vi "Main page.vi"() -> ()   [LabVIEW 2020]
uses:
  Port details.ctl
  SM Cases.ctl
  Control Pages.ctl
  Data Acquisition.ctl
  Array of Port Config.ctl
  Global Data Cluster.ctl
panel:
  out "Proc loop time":dbl
  out "Status":string
  in  "left arrow":bool
  in  "right arrow":bool
  in  "Refresh":bool
  in  "Logout":bool
  out "error out":errorcluster
  in  "Error In":errorcluster
  in  "Instructions":bool
  out "Tab Control":T1(tab)
  out "Success":string
  in  "Confirm":bool
  in  "New Password":string
  in  "Current Password":string
  out "login text":string
  in  "Change password":bool
  in  "Delete User":bool
  in  "View users":bool
  in  "Add user":bool
  in  "Logout user":bool
  in  "Password":string
  in  "Signin":bool
  in  "User Name":string
  in  "Channel2":T2={"Port No."="", "Checkbox"=FALSE, "Parity"=0, "Stop Bit"=0, "Baud Rate"=9600, "Data Bits"=8} {"Stop Bit" items=["1.0", "1.5", "2.0"]; "Parity" items=["None", "Odd", "Even", "Mark", "Space"]}
  in  "Channel1":T3={"Port No."="", "Checkbox"=FALSE, "Parity"=0, "Stop Bit"=0, "Baud Rate"=9600, "Data Bits"=8} {"Stop Bit" items=["1.0", "1.5", "2.0"]; "Parity" items=["None", "Odd", "Even", "Mark", "Space"]}
  in  "Channel8":T2={"Port No."="", "Checkbox"=FALSE, "Parity"=0, "Stop Bit"=0, "Baud Rate"=9600, "Data Bits"=8} {"Stop Bit" items=["1.0", "1.5", "2.0"]; "Parity" items=["None", "Odd", "Even", "Mark", "Space"]}
  in  "Channel7":T2={"Port No."="", "Checkbox"=FALSE, "Parity"=0, "Stop Bit"=0, "Baud Rate"=9600, "Data Bits"=8} {"Stop Bit" items=["1.0", "1.5", "2.0"]; "Parity" items=["None", "Odd", "Even", "Mark", "Space"]}
  in  "Channel6":T2={"Port No."="", "Checkbox"=FALSE, "Parity"=0, "Stop Bit"=0, "Baud Rate"=9600, "Data Bits"=8} {"Stop Bit" items=["1.0", "1.5", "2.0"]; "Parity" items=["None", "Odd", "Even", "Mark", "Space"]}
  in  "Channel5":T2={"Port No."="", "Checkbox"=FALSE, "Parity"=0, "Stop Bit"=0, "Baud Rate"=9600, "Data Bits"=8} {"Stop Bit" items=["1.0", "1.5", "2.0"]; "Parity" items=["None", "Odd", "Even", "Mark", "Space"]}
  in  "Channel4":T2={"Port No."="", "Checkbox"=FALSE, "Parity"=0, "Stop Bit"=0, "Baud Rate"=9600, "Data Bits"=8} {"Stop Bit" items=["1.0", "1.5", "2.0"]; "Parity" items=["None", "Odd", "Even", "Mark", "Space"]}
  in  "Channel3":T2={"Port No."="", "Checkbox"=FALSE, "Parity"=0, "Stop Bit"=0, "Baud Rate"=9600, "Data Bits"=8} {"Stop Bit" items=["1.0", "1.5", "2.0"]; "Parity" items=["None", "Odd", "Even", "Mark", "Space"]}
  in  "Cancel Config":bool
  in  "Save":bool
  in  "Config file view":bool
  out "File Name":string
  in  "Multicolumn Listbox":i32[](listbox)
  in  "Cancel Frame Config":bool
  in  "Save file":bool
  in  "New File":bool
  in  "View data":bool
  in  "Edit structure":bool
  in  "Remove structure":bool
  in  "Add structure":bool
  out "Version":string
  in  "EOH":u8 format="%x"
  in  "No. of bytes":u16 format="%x"
  in  "Message ID":u8 format="%x"
  in  "SOH":u8 format="%x"
  in  "Channel name":u16(ring) items=["Channel1", "Channel2", "Channel3", "Channel4", "Channel5", "Channel6", "Channel7", "Channel8"]
  in  "Cancel Acq":bool
  in  "Stop Acquisition":bool
  in  "Start Acquisition":bool
  in  "FCS Configuration":u16(ring) items=["6012", "7210", "Data_Structure ", "Sim_Struct ", "Sim_Struct_1Port ", "Sim_Struct_3Ports ", "Struct_Channel3 ", "V7352"]
  in  "Port Configuration":u16(ring) items=["LRU_1Port ", "LRU_ch1&2 ", "LRU_ch3&4 ", "LRU_Channel3 ", "LRU_Channel_Config ", "LRU_Config_3Ports ", "LRU_Port_Config "]
  out "% Failure 3":dbl
  out "CRC Failure 3":u32
  out "Frames Read 3":u32
  out "Channel 3":u8(slide) scale=0.0..100.0
  out "% Failure 8":dbl
  out "CRC Failure 8":u32
  out "Frames Read 8":u32
  out "Channel 8":u8(slide) scale=0.0..100.0
  out "% Failure 7":dbl
  out "CRC Failure 7":u32
  out "Frames Read 7":u32
  out "Channel 7":u8(slide) scale=0.0..100.0
  out "% Failure 6":dbl
  out "CRC Failure 6":u32
  out "Frames Read 6":u32
  out "Channel 6":u8(slide) scale=0.0..100.0
  out "% Failure 5":dbl
  out "CRC Failure 5":u32
  out "Frames Read 5":u32
  out "Channel 5":u8(slide) scale=0.0..100.0
  out "% Failure 4":dbl
  out "CRC Failure 4":u32
  out "Frames Read 4":u32
  out "Channel 4":u8(slide) scale=0.0..100.0
  out "% Failure 2":dbl
  out "CRC Failure 2":u32
  out "Frames Read 2":u32
  out "Channel 2":u8(slide) max=150 scale=0.0..100.0
  out "% Failure":dbl
  out "CRC Failure":u32
  out "Frames Read":u32
  out "Channel 1":u8(slide) max=150 scale=0.0..100.0
  in  "Log CRC Failure":enum32{"Log File Yes", "Log File No"}(radio)=enum."Log File No"
  in  "Done":bool
  in  "Refresh":bool
  in  "Update":bool
  in  "Data File Type":enum32{"bin type", "txt type"}(radio)=enum."txt type"
  in  "Data Folder Path":path=path "C:/Users/BEL/Desktop/FCS Rx Data"
  in  "Data Structure Folder Path":path=path "D:/BEL_FCS_Project/FCTS_JIG_LV/Configuration Files/Data Structure"
  in  "Configuration Folder Path":path=path "D:/BEL_FCS_Project/FCTS_JIG_LV/Configuration Files/Port Configuration"
  in  "Help":bool
  in  "Information":bool
  in  "Configuration":bool
  in  "Frame Info":bool
  in  "Frame Format":bool
  in  "Port Configuration":bool
  in  "Authentication":bool
  # "FLIGHT CONTROL SYSTEM\nTEST JIG"
  # "Change Password"
  # "Delete User"
  # "Logout"
  # "Add User"
  # "View Users"
  # "BHARAT ELECTRONICS"
  # "FLIGHT CONTROL SYSTEM (FCS) \nTEST JIG"
  # "COMAVIA SYSTEMS TECHNOLOGIES PRIVATE LIMITED"
  # "VERSION NO."
  # "1.0.0"
  # "RELEASED DATE:"
  # "30/06/2020"
  # "DEVELOPED BY:"
  # "Serial Configuration"
  # "Frame Format"
  # "EOH"
  # "Message ID"
  # "No. of Bytes"
  # "Channel"
  # "SOH"
  # "Frame Info"
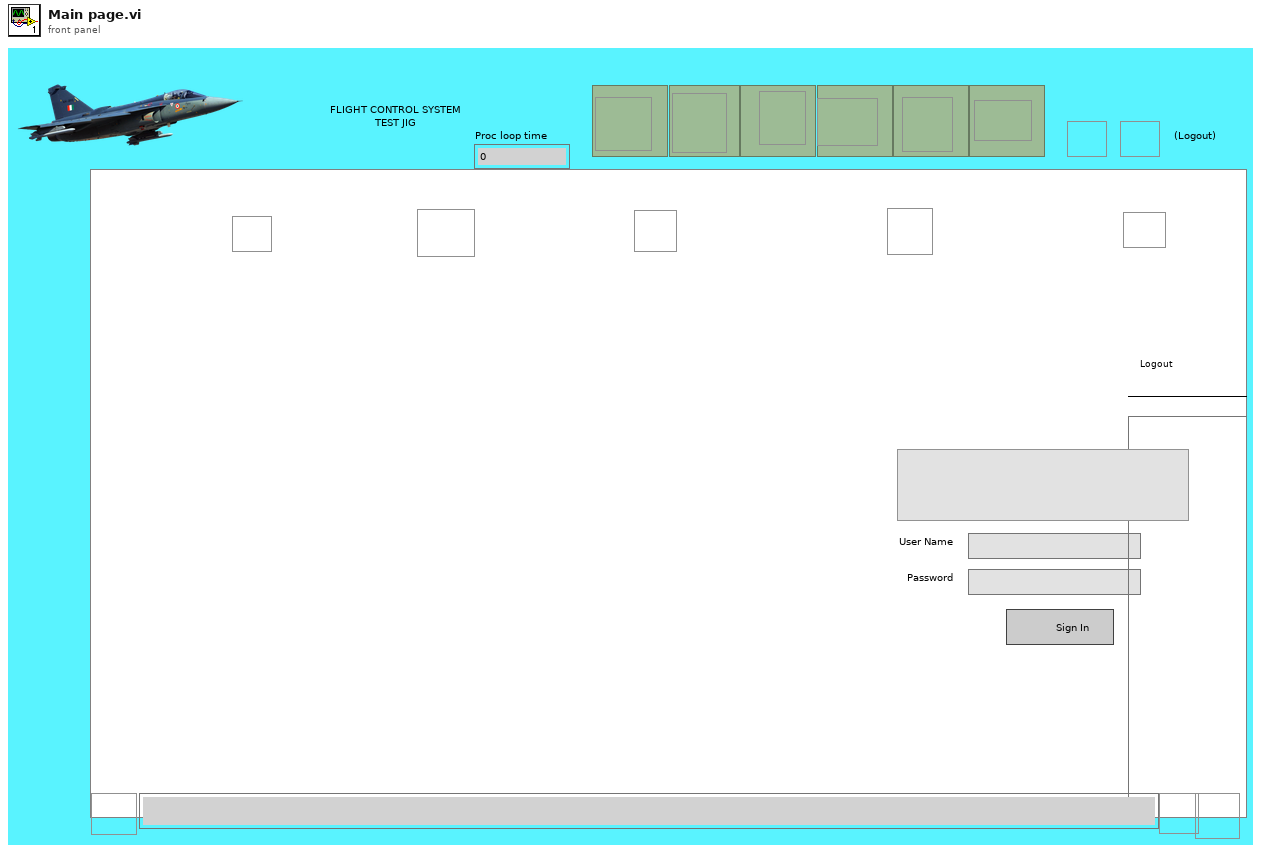
[diagram p1: front panel]
types:
  T1 = enum32{"Authentication", "Home", "Port Config", "Frame Format", "Frame Info", "Configuration", "Page 6", "Page 7"}
  T2 = typedef "Port details.ctl" = cluster{"Port No.":refnum<visa-resource-name>, "Checkbox":bool, "Parity":u16, "Stop Bit":u16, "Baud Rate":u32, "Data Bits":u8}
  T3 = cluster{"Port No.":refnum<visa-resource-name>, "Checkbox":bool, "Parity":u16, "Stop Bit":u16, "Baud Rate":u32, "Data Bits":u8}
  T4 = typedef "SM Cases.ctl" = enum32{"Self-Test", "Initialize", "Poll", "Authentication", "Port Config", "Frame Format", "Frame Info", "Configuration", "User Info", "Logout", "Exit"}
  T5 = typedef "Control Pages.ctl" = enum32{"Authentication", "Home", "Port Config", "Frame Format", "Frame Info", "Configuration", "Page 6", "Page 7"}
  T6 = enum8{"Enabled", "Disabled", "Disabled and Grayed Out"}
  T7 = typedef "Global Data Cluster.ctl" = cluster{"log paths":path[], "CRC paths":path[], "log refnum":refnum<file>[], "CRC refnum":refnum<file>[], "unfiltered array":string[], "Port config":cluster{"data":cluster{"Port No.":refnum<visa-resource-name>, "Checkbox":bool, "Parity":u16, "Stop Bit":u16, "Baud Rate":u32, "Data Bits":u8}[]}, "Filtered array":string[], "Data Structure":string[][]}
  T8 = typedef "Array of Port Config.ctl" = cluster{"Port No.":refnum<visa-resource-name>, "Checkbox":bool, "Parity":u16, "Stop Bit":u16, "Baud Rate":u32, "Data Bits":u8}[]
  T9 = typedef "Data Acquisition.ctl" = enum16{"Port Config", "File Open", "Process Data", "Data Logging", "File Close", "Exit"}
  T10 = enum16{"big-endian, network order", "native, host order", "little-endian"}
  T11 = enum16{"open", "replace", "create", "open or create", "replace or create", "replace or create with confirmation"}
  T12 = cluster{"Port No.":refnum<visa-resource-name>, "Checkbox":bool, "Parity":u16, "Stop Bit":u16, "Baud Rate":u32, "Data Bits":u8}[]
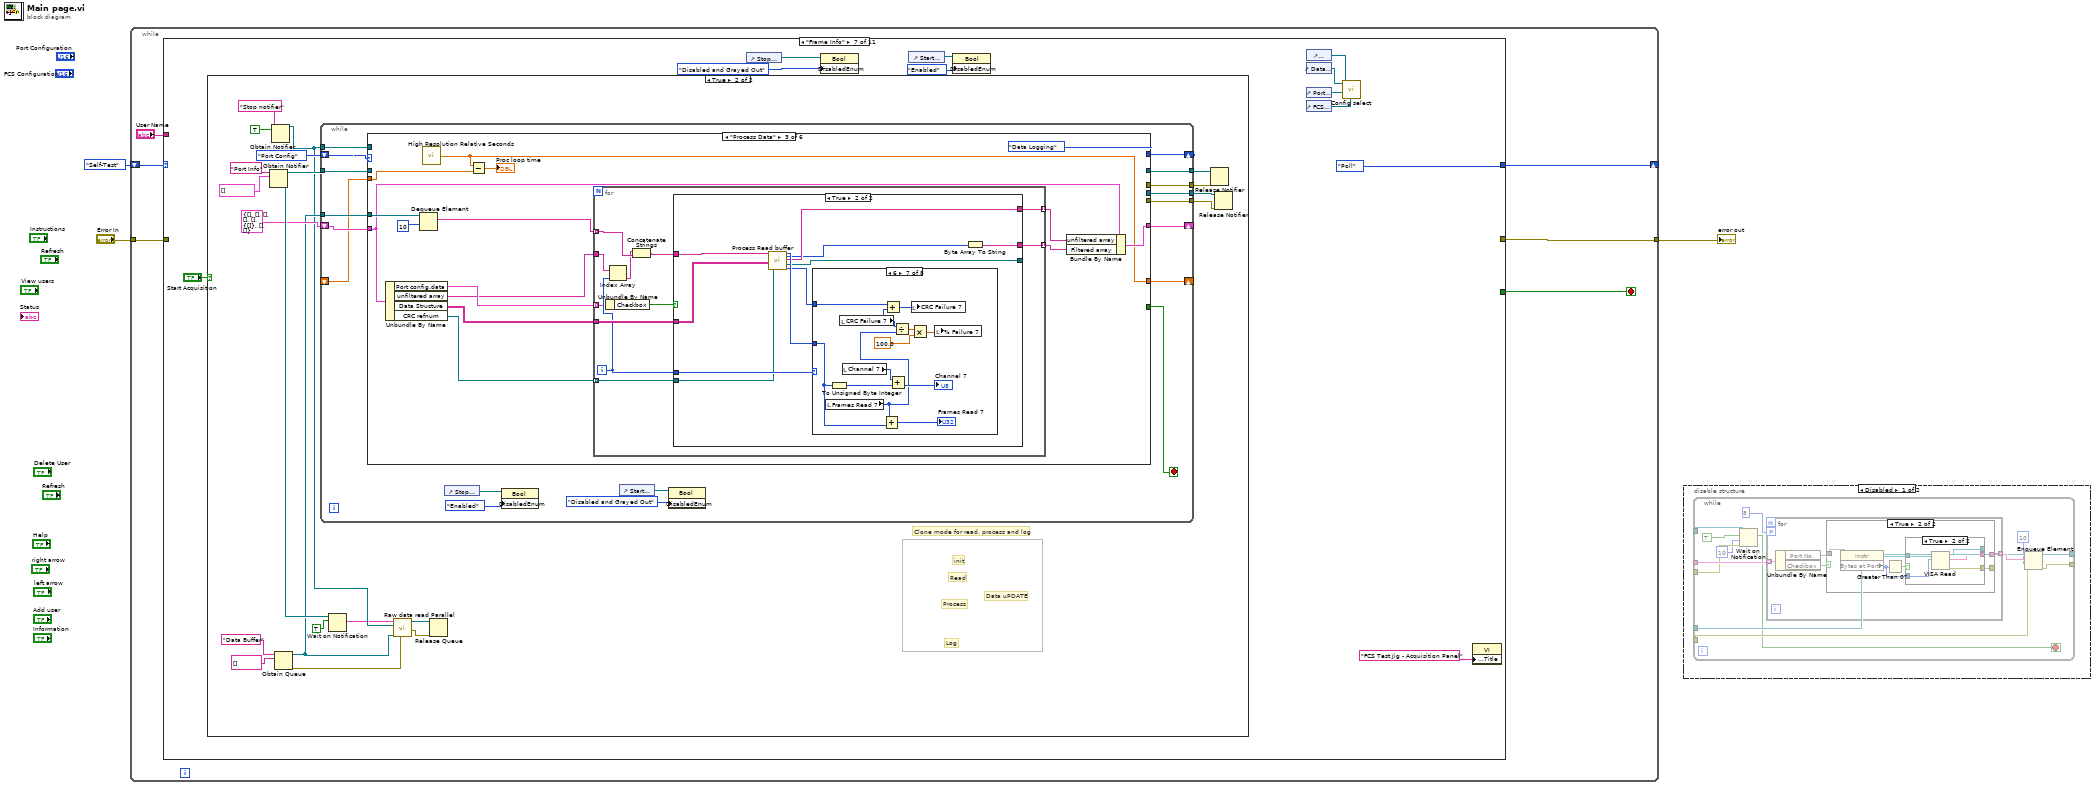
[diagram p0: block diagram]
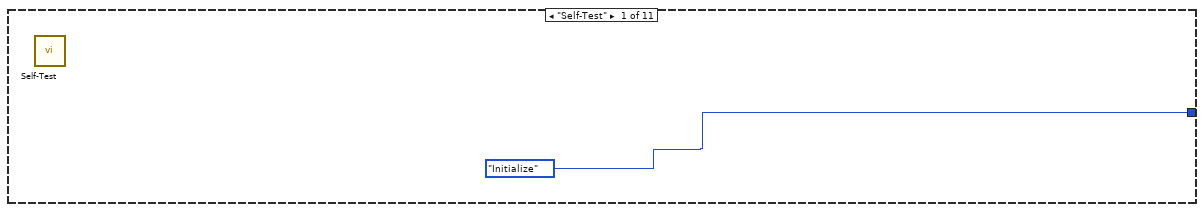
[diagram p5: hidden frame]
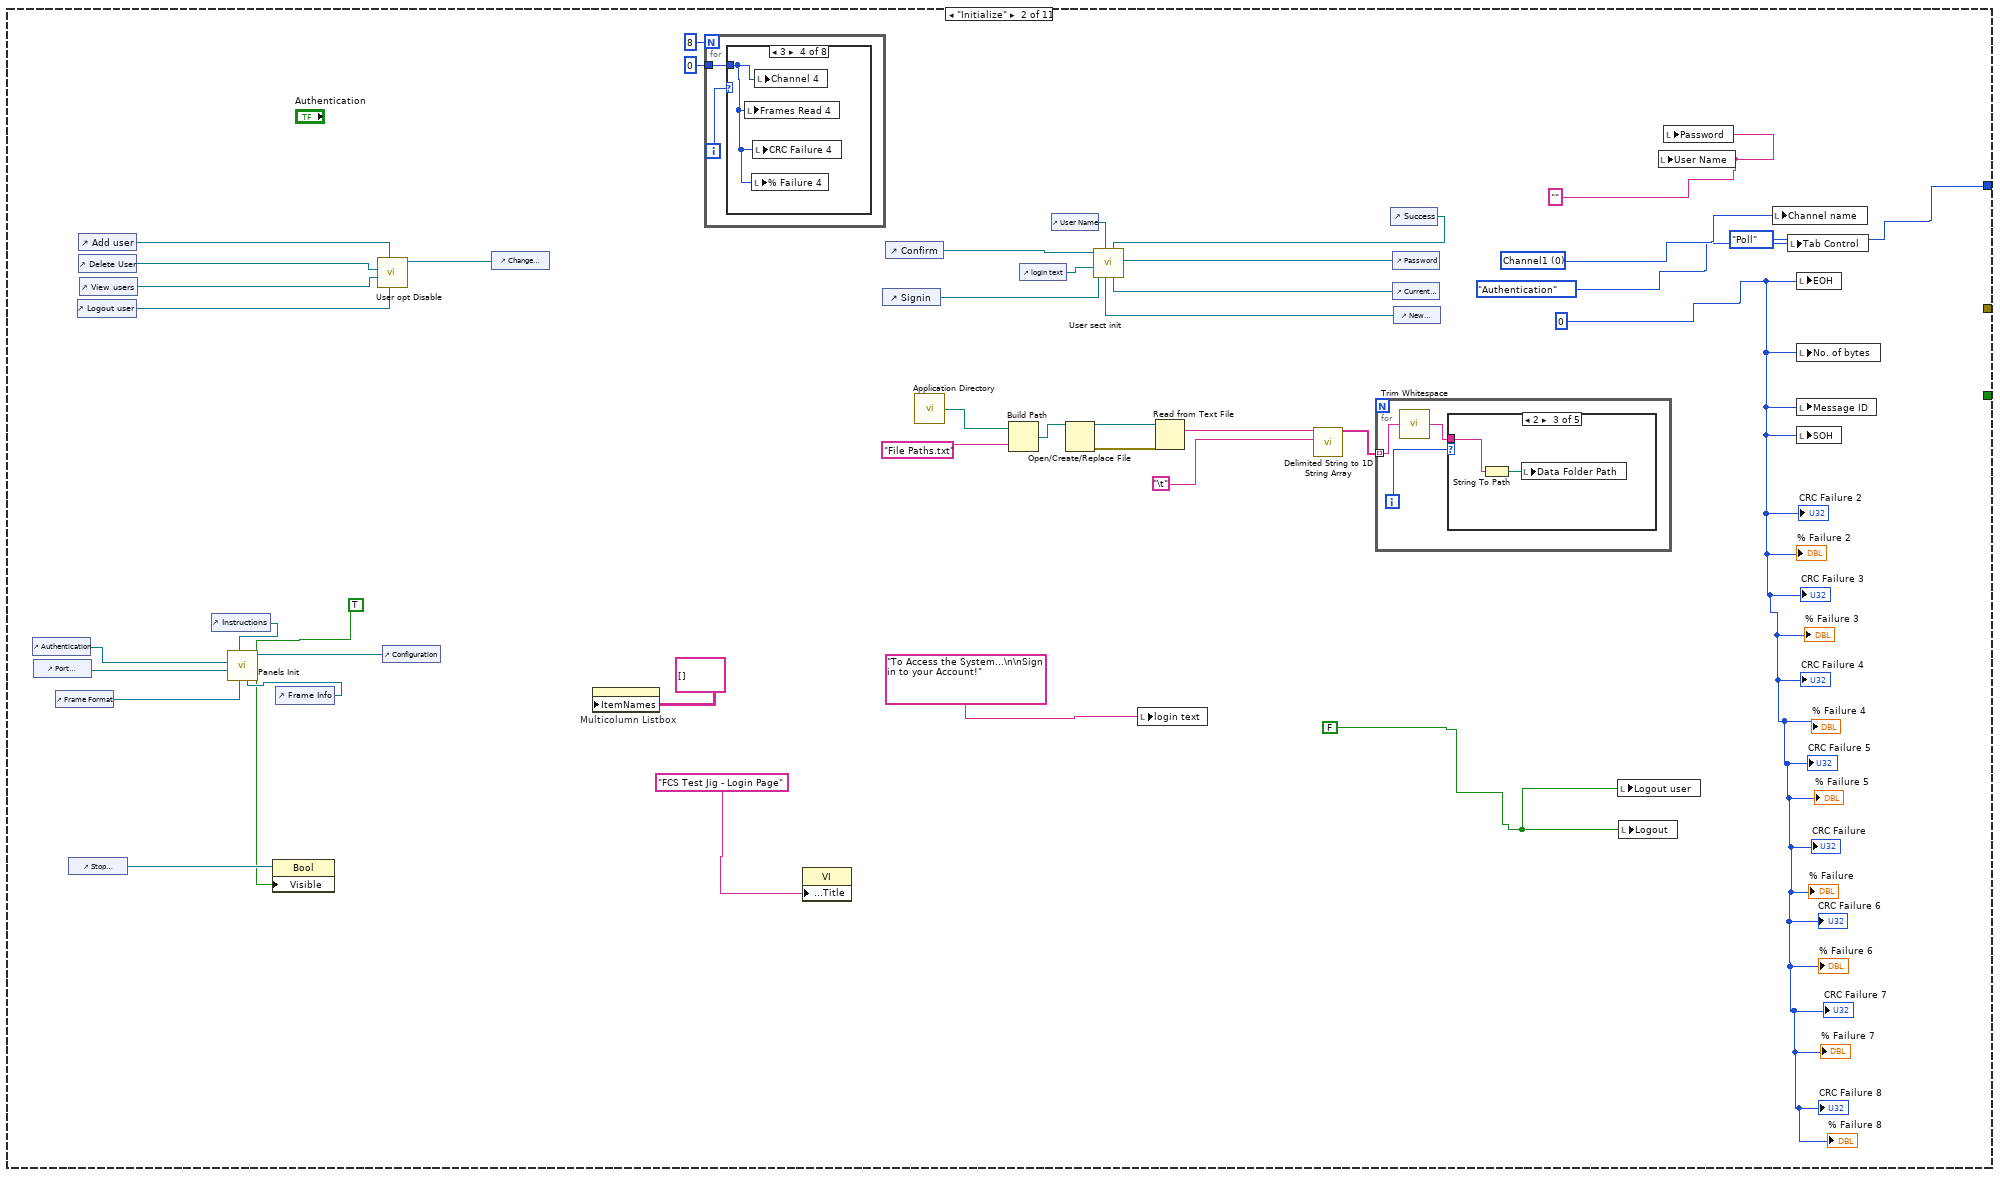
[diagram p6: hidden frame]
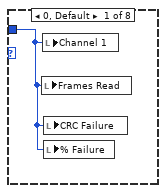
[diagram p7: hidden frame]
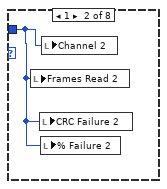
[diagram p8: hidden frame]
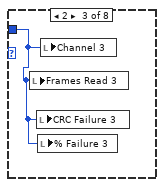
[diagram p9: hidden frame]
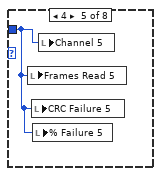
[diagram p10: hidden frame]
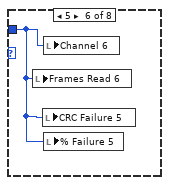
[diagram p11: hidden frame]
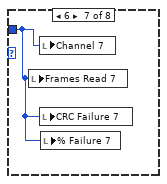
[diagram p12: hidden frame]
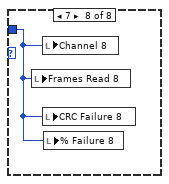
[diagram p13: hidden frame]
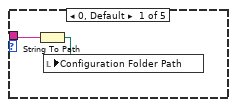
[diagram p14: hidden frame]
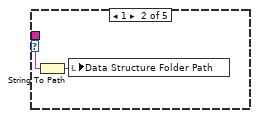
[diagram p15: hidden frame]
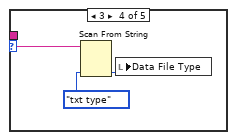
[diagram p16: hidden frame]
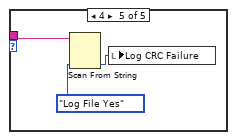
[diagram p17: hidden frame]
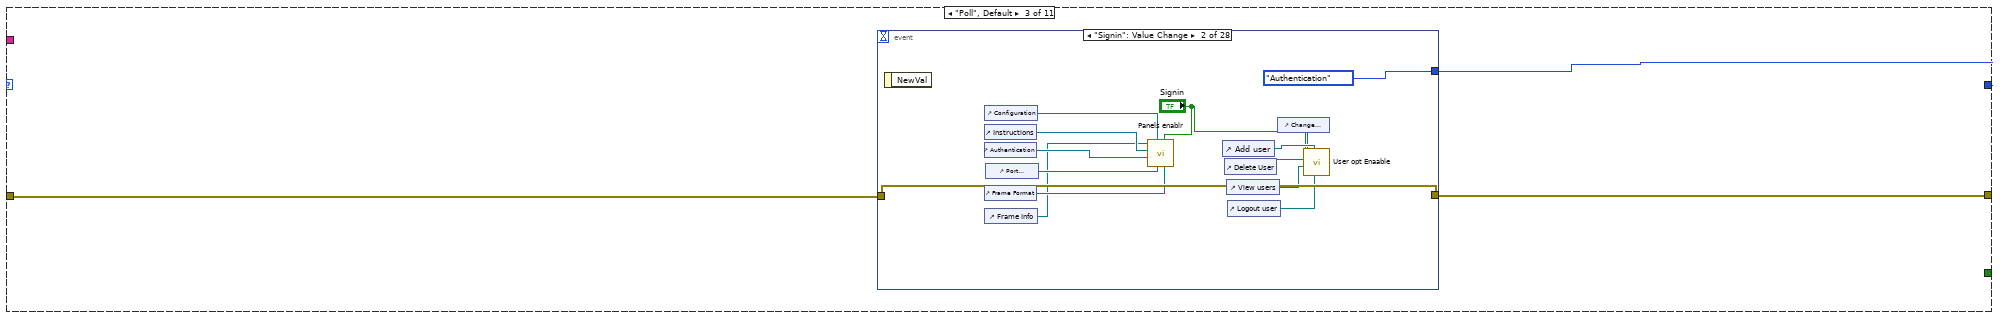
[diagram p18: hidden frame]
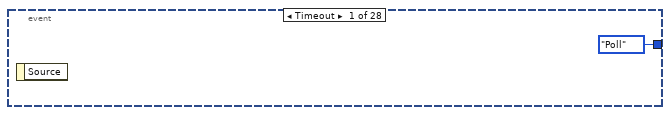
[diagram p19: hidden frame]
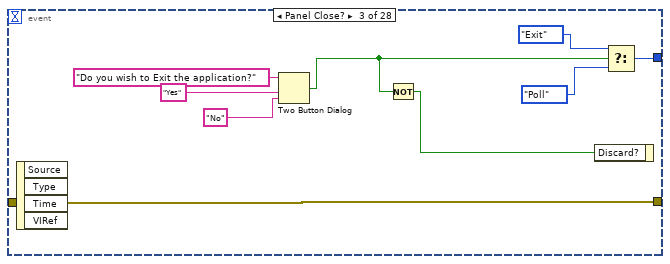
[diagram p20: hidden frame]
diagram:
  n1 = while {
    tunnel: "Error In" -> [w8]
    tunnel: [w7] -> w2
    shift-right: [w6] -> _
    shift-left: SM_Cases."Self-Test" ("Tab Control") -> [w9]
    stop <- w5 stop-if-true
    n2 = case shown="\"Frame Info\"" w9 {
      tunnel: [_ _ w78 w152 _ _ _ _ _ _ _] -> w7
      tunnel: w8 -> [_ _ w77 w153 _ _ _ w567 _ _ _]
      tunnel: [SM_Cases."Initialize" ("Tab Control") SM_Cases."Poll" ("Tab Control") w76 SM_Cases."Poll" ("Tab Control") SM_Cases."Poll" ("Tab Control") SM_Cases."Poll" ("Tab Control") SM_Cases."Poll" ("Tab Control") SM_Cases."Poll" ("Tab Control") SM_Cases."Poll" ("Tab Control") SM_Cases."Initialize" ("Tab Control") SM_Cases."Poll" ("Tab Control")] -> w6
      tunnel: [_ _ _ _ _ _ _ _ _ _ TRUE] -> w5
      tunnel: "User Name" -> [_ _ _ w148 _ _ _ _ _ w629 _]
      frame "Self-Test" {
        n3 = call "Self-Test.vi"() -> ()  [unwired: 12 in]
      }
      frame "Initialize" {
        w11 = FALSE ("Logout")
        w14 = u32 0 ("EOH")
        w49 = u16 0 items=["Channel1", "Channel2", "Channel3", "Channel4", "Channel5", "Channel6", "Channel7", "Channel8"] ("Ring")
        w29 = "" ("Password")
        n4 = control-ref of="Authentication"() -> (w41:refnum<vi>)
        n5 = control-ref of="Port Configuration"() -> (w40:refnum<vi>)
        n6 = control-ref of="Frame Format"() -> (w39:refnum<vi>)
        n7 = control-ref of="Stop Acquisition"() -> (w24:refnum<vi>)
        n8 = control-ref of="Logout user"() -> (w32:refnum<vi>)
        n9 = control-ref of="Add user"() -> (w33:refnum<vi>)
        n10 = control-ref of="Delete User"() -> (w34:refnum<vi>)
        n11 = control-ref of="View users"() -> (w35:refnum<vi>)
        n12 = control-ref of="Instructions"() -> (w36:refnum<vi>)
        n13 = property class="Bool"(reference=w24, "Visible"=TRUE) -> ()  [unwired: 1 in, 2 out]
        n14 = control-ref of="Frame Info"() -> (w38:refnum<vi>)
        n15 = control-ref of="Configuration"() -> (w37:refnum<vi>)
        n16 = call "Panels Init.vi"("Frame Info"=w38, "Frame Format"=w39, "Instructions"=w36, "Port Configuration"=w40, "Authentication"=w41, "Boolean in"=w37) -> ()  [unwired: 6 in]
        n17 = control-ref of="Change password"() -> (w31:refnum<vi>)
        n18 = call "User opt Disable.vi"("Logout user"=w32, "Add user"=w33, "View users"=w35, "Delete User"=w34, "Boolean in"=w31) -> ()  [unwired: 7 in]
        n19 = property on="Multicolumn Listbox" class="MCListbox (strict)"("ItemNames"=string[][] [] ("Item Names")) -> ()  [unwired: 2 in, 2 out]
        n20 = for {
          N: 8 -> [_]
          tunnel: u32 0 -> [w52]
          i -> [w51]
          n21 = case shown="3" w51 {
            tunnel: w52 -> [w53 w54 w55 w56 w57 w58 w59 w60]
            frame 0, Default {
              n22 = local write "Frames Read"(w53) -> ()
              n23 = local write "Channel 1"(w53) -> ()
              n24 = local write "CRC Failure"(w53) -> ()
              n25 = local write "% Failure"(w53) -> ()
            }
            frame 1 {
              n26 = local write "Frames Read 2"(w54) -> ()
              n27 = local write "CRC Failure 2"(w54) -> ()
              n28 = local write "% Failure 2"(w54) -> ()
              n29 = local write "Channel 2"(w54) -> ()
            }
            frame 2 {
              n30 = local write "Frames Read 3"(w55) -> ()
              n31 = local write "CRC Failure 3"(w55) -> ()
              n32 = local write "% Failure 3"(w55) -> ()
              n33 = local write "Channel 3"(w55) -> ()
            }
            frame 3 {
              n34 = local write "Frames Read 4"(w56) -> ()
              n35 = local write "% Failure 4"(w56) -> ()
              n36 = local write "CRC Failure 4"(w56) -> ()
              n37 = local write "Channel 4"(w56) -> ()
            }
            frame 4 {
              n38 = local write "Frames Read 5"(w57) -> ()
              n39 = local write "CRC Failure 5"(w57) -> ()
              n40 = local write "% Failure 5"(w57) -> ()
              n41 = local write "Channel 5"(w57) -> ()
            }
            frame 5 {
              n42 = local write "Frames Read 6"(w58) -> ()
              n43 = local write "CRC Failure 5"(w58) -> ()
              n44 = local write "Channel 6"(w58) -> ()
              n45 = local write "% Failure 5"(w58) -> ()
            }
            frame 6 {
              n46 = local write "Frames Read 7"(w59) -> ()
              n47 = local write "Channel 7"(w59) -> ()
              n48 = local write "CRC Failure 7"(w59) -> ()
              n49 = local write "% Failure 7"(w59) -> ()
            }
            frame 7 {
              n50 = local write "Frames Read 8"(w60) -> ()
              n51 = local write "Channel 8"(w60) -> ()
              n52 = local write "CRC Failure 8"(w60) -> ()
              n53 = local write "% Failure 8"(w60) -> ()
            }
          }
        }
        n54 = property class="VI"("Front Panel.Title"="FCS Test Jig - Login Page" ("VI Name")) -> ()  [unwired: 2 in, 2 out]
        n55 = control-ref of="Signin"() -> (w46:refnum<vi>)
        n56 = control-ref of="Confirm"() -> (w44:refnum<vi>)
        n57 = call <vilib>:"Application Directory.vi"() -> ("Application Directory"=w22:path)
        n58 = Build Path(base path=w22, name or relative path="File Paths.txt") -> (appended path=w20:path)
        n59 = control-ref of="login text"() -> (w47:refnum<vi>)
        n60 = control-ref of="User Name"() -> (w28:refnum<vi>)
        n61 = Open/Create/Replace File(file path (use dialog)=w20) -> (refnum out=w18:refnum<file>, error out=w19:errorcluster)  [unwired: 5 in, 1 out]
        n62 = local write "login text"("To Access the System...\n\nSign in to your Account!" ("login text")) -> ()
        n63 = Read from Text File(file (use dialog)=w18, error in=w19) -> (text=w17:string)  [unwired: 2 in, 3 out]
        n64 = call <vilib>:"Delimited String to 1D String Array.vi"("delimiter"="\t", "delimited string"=w17) -> ("string array"=w15:string[])  [unwired: 9 in]
        n65 = for {
          tunnel: w15 -> [w62] mode=indexing
          i -> [w63]
          n66 = call <vilib>:"Trim Whitespace.vi"("string"=w62) -> ("trimmed string"=w61:string)  [unwired: 1 in]
          n67 = case shown="2" w63 {
            tunnel: w61 -> [w65 w67 w69 w72 w75]
            frame 0, Default {
              n68 = String To Path(string=w65) -> (path=w64:path)
              n69 = local write "Configuration Folder Path"(w64) -> ()
            }
            frame 1 {
              n70 = String To Path(string=w67) -> (path=w66:path)
              n71 = local write "Data Structure Folder Path"(w66) -> ()
            }
            frame 2 {
              n72 = String To Path(string=w69) -> (path=w68:path)
              n73 = local write "Data Folder Path"(w68) -> ()
            }
            frame 3 {
              n74 = Scan From String(input string=w72, default 1=enum32{"bin type", "txt type"}."txt type" ("Data File Type")) -> (output 1=w70:enum32{"bin type", "txt type"})  [unwired: 3 in, 3 out]
              n75 = local write "Data File Type"(w70) -> ()
            }
            frame 4 {
              n76 = Scan From String(input string=w75, default 1=enum32{"Log File Yes", "Log File No"}."Log File Yes" ("Log CRC Failure")) -> (output 1=w73:enum32{"Log File Yes", "Log File No"})  [unwired: 3 in, 3 out]
              n77 = local write "Log CRC Failure"(w73) -> ()
            }
          }
        }
        n78 = control-ref of="Success"() -> (w42:refnum<vi>)
        n79 = control-ref of="Password"() -> (w48:refnum<vi>)
        n80 = control-ref of="Current Password"() -> (w45:refnum<vi>)
        n81 = control-ref of="New Password"() -> (w43:refnum<vi>)
        n82 = call "User sect init.vi"("Current Password"=w45, "Success"=w42, "New Password"=w43, "User Name"=w28, "Signin"=w46, "login text"=w47, "Password"=w48, "Boolean in"=w44) -> ()  [unwired: 4 in]
        n83 = local write "Logout user"(w11) -> ()
        n84 = local write "Logout"(w11) -> ()
        n85 = local write "User Name"(w29) -> ()
        n86 = local write "Password"(w29) -> ()
        n87 = local write "Channel name"(w49) -> ()
        n88 = local write "Tab Control"(Control_Pages."Authentication" ("Tab Control")) -> ()
        n89 = local write "EOH"(w14) -> ()
        n90 = local write "No. of bytes"(w14) -> ()
        n91 = local write "Message ID"(w14) -> ()
        n92 = local write "SOH"(w14) -> ()
        "CRC Failure 2" <- w14
        "% Failure 2" <- w14
        "CRC Failure 3" <- w14
        "% Failure 3" <- w14
        "CRC Failure 4" <- w14
        "% Failure 4" <- w14
        "CRC Failure 5" <- w14
        "% Failure 5" <- w14
        "CRC Failure 6" <- w14
        "% Failure 6" <- w14
        "CRC Failure 7" <- w14
        "% Failure 7" <- w14
        "CRC Failure 8" <- w14
        "% Failure 8" <- w14
        "CRC Failure" <- w14
        "% Failure" <- w14
      }
      frame "Poll", Default {
        n93 = event shown="[1] \"Signin\": Value Change" {
          selector: _ -> [_ _ _ _ _ _ _ _ _ _ _ _ _ _ _ _ _ _ _ _ _ _ _ _ _ _ _ _]
          dyn-events: _ -> [_ _ _ _ _ _ _ _ _ _ _ _ _ _ _ _ _ _ _ _ _ _ _ _ _ _ _ _]
          timeout: _ -> [_ _ _ _ _ _ _ _ _ _ _ _ _ _ _ _ _ _ _ _ _ _ _ _ _ _ _ _]
          tunnel: [_ w93 w102 _ _ _ _ _ _ _ _ _ _ _ _ _ _ _ _ _ _ _ _ _ _ _ _ _] -> w78
          tunnel: w77 -> [_ w93 w102 _ _ _ _ _ _ _ _ _ _ _ _ _ _ _ _ _ _ _ _ _ _ _ _ _]
          tunnel: [SM_Cases."Poll" ("Tab Control") SM_Cases."Authentication" ("Tab Control") w97 SM_Cases."Frame Format" ("Tab Control") SM_Cases."Port Config" ("Tab Control") SM_Cases."Frame Info" ("Tab Control") SM_Cases."User Info" ("Tab Control") SM_Cases."Logout" ("Tab Control") SM_Cases."User Info" ("Tab Control") SM_Cases."User Info" ("Tab Control") SM_Cases."Logout" ("Tab Control") SM_Cases."Port Config" ("Tab Control") SM_Cases."Configuration" ("Tab Control") SM_Cases."Configuration" ("Tab Control") SM_Cases."Frame Format" ("Tab Control") SM_Cases."Frame Format" ("Tab Control") SM_Cases."Frame Format" ("Tab Control") SM_Cases."Frame Format" ("Tab Control") SM_Cases."Poll" ("Tab Control") SM_Cases."Port Config" ("Tab Control") SM_Cases."Frame Format" ("Tab Control") SM_Cases."Frame Format" ("Tab Control") SM_Cases."Poll" ("Tab Control") SM_Cases."Port Config" ("Tab Control") SM_Cases."Frame Format" ("Tab Control") SM_Cases."Frame Info" ("Tab Control") SM_Cases."Frame Info" ("Tab Control") SM_Cases."Configuration" ("Tab Control")] -> w76
          event Timeout {
            n94 = event-data() -> ()  [unwired: 1 in, 1 out]
          }
          event "Signin": Value Change {
            n95 = event-data() -> ()  [unwired: 1 in, 1 out]
            n96 = control-ref of="Instructions"() -> (w90:refnum<vi>)
            n97 = control-ref of="Authentication"() -> (w89:refnum<vi>)
            n98 = control-ref of="Frame Format"() -> (w87:refnum<vi>)
            n99 = control-ref of="Configuration"() -> (w91:refnum<vi>)
            n100 = control-ref of="Frame Info"() -> (w86:refnum<vi>)
            n101 = control-ref of="Port Configuration"() -> (w88:refnum<vi>)
            n102 = call "Panels enablr.vi"("Frame Format"=w87, "Signin"="Signin", "Port Configuration"=w88, "Configuration"=w91, "Authentication"=w89, "Instructions"=w90, "Boolean in"=w86) -> ()  [unwired: 5 in]
            n103 = control-ref of="Add user"() -> (w85:refnum<vi>)
            n104 = control-ref of="Delete User"() -> (w84:refnum<vi>)
            n105 = control-ref of="View users"() -> (w83:refnum<vi>)
            n106 = control-ref of="Logout user"() -> (w82:refnum<vi>)
            n107 = control-ref of="Change password"() -> (w81:refnum<vi>)
            n108 = call "User opt Enaable.vi"("Logout user"=w82, "Add user"=w85, "Boolean"="Signin", "View users"=w83, "Delete User"=w84, "Boolean in"=w81) -> ()  [unwired: 6 in]
          }
          event Panel Close? {
            n109 = event-data() -> ()  [unwired: 1 in, 4 out]
            n110 = Two Button Dialog(message="Do you wish to Exit the application?", 1:"No" ("F button name (\"Cancel\")"), 2:"Yes" ("T button name (\"OK\")")) -> (T button?=w95:bool)
            n111 = Not(x=w95) -> (.not. x?=w94:bool)
            n112 = event-data("Discard?"=w94) -> ()  [unwired: 1 in, 1 out]
            n113 = Select(t=SM_Cases."Exit" ("Tab Control"), s=w95, f=SM_Cases."Poll" ("Tab Control")) -> (s? t:f=w97:T4)
          }
          event "Frame Format": Value Change {
            n114 = event-data() -> ()  [unwired: 1 in, 1 out]
            n115 = local write "Tab Control"(T1."Frame Format" ("Tab Control")) -> ()
            n116 = local write "No. of bytes"(u16 1 ("No. of bytes")) -> ()
            n117 = local write "Message ID"(u8 1 ("Message ID")) -> ()
            n118 = local write "SOH"(u8 1 ("SOH")) -> ()
            n119 = local write "EOH"(u8 1 ("EOH")) -> ()
          }
          event "Port Configuration": Value Change {
            n120 = event-data() -> ()  [unwired: 1 in, 1 out]
            n121 = local write "Tab Control"(T1."Port Config" ("Tab Control")) -> ()
          }
          event "Frame Info": Value Change {
            n122 = event-data() -> ()  [unwired: 1 in, 1 out]
            n123 = local write "Tab Control"(T1."Frame Info" ("Tab Control")) -> ()
          }
          event "Authentication": Value Change {
            n124 = event-data() -> ()  [unwired: 1 in, 1 out]
            n125 = property class="VI"("Front Panel.Title"="FCS Test Jig - Access Panel" ("VI Name")) -> ()  [unwired: 2 in, 2 out]
            "Tab Control" <- T1."Authentication" ("Tab Control")
          }
          event "Logout user": Value Change {
            n126 = event-data() -> ()  [unwired: 1 in, 6 out]
          }
          event "Change password": Value Change {
            n127 = event-data() -> ()  [unwired: 1 in, 1 out]
          }
          event "Confirm": Value Change {
            n128 = event-data() -> ()  [unwired: 1 in, 6 out]
          }
          event "Logout": Value Change {
            n129 = event-data() -> ()  [unwired: 1 in, 6 out]
          }
          event "Save": Value Change {
            n130 = event-data() -> ()  [unwired: 1 in, 6 out]
          }
          event "Configuration": Value Change {
            n131 = event-data() -> ()  [unwired: 1 in, 6 out]
            n132 = local write "Tab Control"(T1."Configuration" ("Tab Control")) -> ()
          }
          event "Done": Value Change {
            n133 = event-data() -> ()  [unwired: 1 in, 6 out]
          }
          event "Add structure": Value Change {
            n134 = event-data() -> ()  [unwired: 1 in, 6 out]
          }
          event "Remove structure": Value Change {
            n135 = event-data() -> ()  [unwired: 1 in, 1 out]
          }
          event "Edit structure": Value Change {
            n136 = event-data() -> ()  [unwired: 1 in, 6 out]
          }
          event "Save file": Value Change {
            n137 = event-data() -> ()  [unwired: 1 in, 6 out]
          }
          event "Multicolumn Listbox": Double Click {
            n138 = event-data() -> ("Row"=w128:i32)  [unwired: 1 in]
            n139 = control-ref of="Multicolumn Listbox"() -> (w129:refnum<vi>)
            n140 = control-ref of="SOH"() -> (w133:refnum<vi>)
            n141 = control-ref of="Message ID"() -> (w132:refnum<vi>)
            n142 = control-ref of="No. of bytes"() -> (w131:refnum<vi>)
            n143 = control-ref of="EOH"() -> (w130:refnum<vi>)
            n144 = control-ref of="Channel name"() -> (w134:refnum<vi>)
            n145 = call "Structure Data Change.vi"("reference 5"=w130, "Row"=w128, "reference 4"=w131, "reference"=w134, "reference 3"=w132, "reference 2"=w133, "MCListbox Refnum"=w129) -> ()  [unwired: 5 in]
          }
          event "Config file view": Value Change {
            n146 = event-data() -> ()  [unwired: 1 in, 6 out]
          }
          event "View data": Value Change {
            n147 = event-data() -> ()  [unwired: 1 in, 6 out]
          }
          event "New File": Value Change {
            n148 = event-data() -> ()  [unwired: 1 in, 6 out]
          }
          event "Cancel Acq": Value Change {
            n149 = event-data() -> ()  [unwired: 1 in, 6 out]
            n150 = case shown="True" "Cancel Acq" {
              frame False {
              }
              frame True {
                n151 = local write "Tab Control"(T1."Home" ("Tab Control")) -> ()
                n152 = property class="VI"("Front Panel.Title"="FCS Test Jig - Home Page" ("VI Name")) -> ()  [unwired: 2 in, 2 out]
              }
            }
          }
          event "Cancel Config": Value Change {
            n153 = event-data() -> ()  [unwired: 1 in, 6 out]
          }
          event "Cancel Frame Config": Value Change {
            n154 = event-data() -> ()  [unwired: 1 in, 6 out]
          }
          event "Start Acquisition": Value Change {
            n155 = event-data() -> ()  [unwired: 1 in, 6 out]
          }
          event "Stop Acquisition": Value Change {
            n156 = event-data() -> ()  [unwired: 1 in, 6 out]
          }
          event "Update": Value Change {
            n157 = event-data() -> ()  [unwired: 1 in, 6 out]
          }
        }
      }
      frame "Authentication" {
        n158 = control-ref of="Tab Control"() -> (w150:refnum<vi>)
        n159 = control-ref of="Status"() -> (w151:refnum<vi>)
        n160 = call "User Authentication.vi"("User Name"=w148, "error in (no error)"=w153, "Password"="Password", "Status"=w151, "TabControl in"=w150) -> ("error out"=w152:errorcluster, "login text"=→"login text":string)  [unwired: 5 in]
      }
      frame "Port Config" {
        n161 = control-ref of="Channel7"() -> (w160:refnum<vi>)
        n162 = control-ref of="Channel2"() -> (w163:refnum<vi>)
        n163 = control-ref of="Channel8"() -> (w161:refnum<vi>)
        n164 = control-ref of="Configuration Folder Path"() -> (w164:refnum<vi>)
        n165 = control-ref of="Channel3"() -> (w162:refnum<vi>)
        n166 = control-ref of="Channel4"() -> (w159:refnum<vi>)
        n167 = control-ref of="Status"() -> (w179:refnum<vi>)
        n168 = local read "Configuration Folder Path"() -> (w178:path)
        n169 = call "Config File Save.vi"("String in"=w179, "Channel 5"="Channel5", "Channel 6"="Channel6", "Channel 7"="Channel7", "Channel 8"="Channel8", "Channel 1"="Channel1", "Configuration Folder Path"=w178, "Channel 4"="Channel4", "Channel 2"="Channel2", "Channel 3"="Channel3", "Save"="Save") -> ("File Name"=w168:string)  [unwired: 4 in]
        n170 = local write "File Name"(w168) -> ()
        n171 = control-ref of="Channel1"() -> (w166:refnum<vi>)
        n172 = control-ref of="Channel5"() -> (w158:refnum<vi>)
        n173 = control-ref of="Channel6"() -> (w157:refnum<vi>)
        n174 = call "File View SubVI.vi"("Channel 8"=w161, "Channel 1"=w166, "Config Path"=w164, "Config file view"="Config file view", "Channel 7"=w160, "Channel 2"=w163, "Channel 3"=w162, "Channel 4"=w159, "Channel 5"=w158, "Channel 6"=w157) -> ("File Name"=→"File Name":string)  [unwired: 5 in]
        n175 = case shown="True" "Cancel Config" {
          frame False {
          }
          frame True {
            n176 = local write "Tab Control"(T1."Home" ("Tab Control")) -> ()
            n177 = property class="VI"("Front Panel.Title"="FCS Test Jig - Home Page" ("VI Name")) -> ()  [unwired: 2 in, 2 out]
          }
        }
        n178 = property class="VI"("Front Panel.Title"="FCS Test Jig - Configuration Panel" ("VI Name")) -> ()  [unwired: 2 in, 2 out]
      }
      frame "Frame Format" {
        n179 = control-ref of="Multicolumn Listbox"() -> (w201:refnum<vi>)
        n180 = local read "Message ID"() -> (w198:u8)
        n181 = case shown="True" "New File" {
          frame False {
          }
          frame True {
            n182 = Initialize Array("") -> (w214:string[][])  [unwired: 2 in]
            n183 = property on="Multicolumn Listbox" class="MCListbox (strict)"("ItemNames"=w214) -> ()  [unwired: 2 in, 2 out]
          }
        }
        n184 = call "Add Structure.vi"("EOH"="EOH", "No. of bytes"="No. of bytes", 7:"Channel name", "MCListbox Refnum"=w201, "Message ID"="Message ID", "Add structure"="Add structure", "SOH"="SOH") -> ()  [unwired: 5 in]
        n185 = local read "Channel name"() -> (w199:u16)
        n186 = local read "SOH"() -> (w197:u8)
        n187 = call "Remove Structure.vi"("Remove structure"="Remove structure", "MCListbox in"=w201, "Array"="Multicolumn Listbox") -> ()  [unwired: 8 in, 1 out]
        n188 = local read "No. of bytes"() -> (w196:u16)
        n189 = local read "EOH"() -> (w195:u8)
        n190 = call "Edit Structure.vi"("EOH"=w195, "Edit structure"="Edit structure", "No. of Bytes"=w196, "Channel ID"=w199, "Message ID"=w198, "SOH"=w197, "MulticolumnListbox in"=w201) -> ()  [unwired: 5 in]
        n191 = control-ref of="Multicolumn Listbox"() -> (w185:refnum<vi>)
        n192 = control-ref of="Data Structure Folder Path"() -> (w194:refnum<vi>)
        n193 = control-ref of="Status"() -> (w187:refnum<vi>)
        n194 = control-ref of="Multicolumn Listbox"() -> (w191:refnum<vi>)
        n195 = case shown="True" "Cancel Frame Config" {
          frame False {
          }
          frame True {
            n196 = local write "Tab Control"(T1."Home" ("Tab Control")) -> ()
            n197 = property class="VI"("Front Panel.Title"="FCS Test Jig - Home Page" ("VI Name")) -> ()  [unwired: 2 in, 2 out]
          }
        }
        n198 = call "Save Structure.vi"("Status Refnum"=w187, "Save file"="Save file", "MCListbox Refnum"=w185, "Path in"=w194) -> ("File Name"=w188:string)  [unwired: 7 in]
        n199 = control-ref of="Data Structure Folder Path"() -> (w192:refnum<vi>)
        n200 = call "View Structure.vi"("View data"="View data", "MCListbox Refnum"=w191, "Path in"=w192) -> ("Version"=→"Version":string)  [unwired: 8 in]
        n201 = local write "Version"(w188) -> ()
        n202 = property class="VI"("Front Panel.Title"="FCS Test Jig - Data Strucuture Panel" ("VI Name")) -> ()  [unwired: 2 in, 2 out]
      }
      frame "Frame Info" {
        n203 = case shown="True" "Start Acquisition" {
          frame False {
          }
          frame True {
            # "Clone mode for read, process and log"
            # "Data uPDATE"
            # "init"
            # "Log"
            # "Process"
            # "Read"
            n204 = Obtain Notifier(name (unnamed)="Port Info", notification data type=T8 [] ("Array")) -> (notifier out=w244:refnum<notifier>)  [unwired: 2 in, 2 out]
            n205 = Obtain Notifier(name (unnamed)="Stop notifier", notification data type=TRUE) -> (notifier out=w231:refnum<notifier>)  [unwired: 2 in, 2 out]
            n206 = Obtain Queue(name (unnamed)="Data Buffer", element data type=string[] []) -> (queue out=w232:refnum<queue>, error out=w229:errorcluster)  [unwired: 3 in, 1 out]
            n207 = while {
              shift-right: [w260] -> _
              shift-left: Data_Acquisition."Port Config" -> [w259]
              tunnel: w244 -> [w258]
              tunnel: [w257] -> w243
              tunnel: [w256] -> w241
              tunnel: w232 -> [w255]
              tunnel: w231 -> [w253]
              tunnel: [w252] -> w237
              tunnel: [w251] -> w236
              shift-right: [w250] -> _
              shift-left: T7 {"log paths"=[], "CRC paths"=[], "log refnum"=[], "CRC refnum"=[], "unfiltered array"=[], "Port config"={"data"=[]}, "Filtered array"=[], "Data Structure"=[]} -> [w249]
              shift-right: [w248] -> _
              shift-left: _ -> [w247]
              stop <- w254 stop-if-true
              n208 = case shown="\"Process Data\"" w259 {
                tunnel: [_ _ _ _ _ TRUE] -> w254
                tunnel: [Data_Acquisition."File Open" Data_Acquisition."Process Data" Data_Acquisition."Data Logging" Data_Acquisition."File Close" w535 _] -> w260
                tunnel: w258 -> [w279 _ _ _ _ w556]
                tunnel: [w278 _ _ _ _ w556] -> w257
                tunnel: [w277 _ _ _ _ _] -> w256
                tunnel: w255 -> [_ _ w371 _ _ _]
                tunnel: w253 -> [_ _ _ _ w533 w554]
                tunnel: [_ _ _ _ w531 w554] -> w252
                tunnel: [_ _ _ _ w530 _] -> w251
                tunnel: w249 -> [w272 w292 w367 w493 w525 w553]
                tunnel: [w270 w291 w364 w493 w525 w553] -> w250
                tunnel: [w265 _ w362 w492 w523 _] -> w248
                tunnel: w247 -> [w265 _ w361 w492 w523 _]
                frame "Port Config", Default {
                  n209 = for {
                    N: 8 -> [_]
                    tunnel: u32 0 -> [w282]
                    i -> [w281]
                    n210 = case shown="0, Default" w281 {
                      tunnel: w282 -> [w283 w284 w285 w286 w287 w288 w289 w290]
                      frame 0, Default {
                        n211 = local write "Channel 1"(w283) -> ()
                        n212 = local write "CRC Failure"(w283) -> ()
                        n213 = local write "% Failure"(w283) -> ()
                        n214 = local write "Frames Read"(w283) -> ()
                      }
                      frame 1 {
                        n215 = local write "Channel 2"(w284) -> ()
                        n216 = local write "Frames Read 2"(w284) -> ()
                        n217 = local write "CRC Failure 2"(w284) -> ()
                        n218 = local write "% Failure 2"(w284) -> ()
                      }
                      frame 2 {
                        n219 = local write "Channel 3"(w285) -> ()
                        n220 = local write "Frames Read 3"(w285) -> ()
                        n221 = local write "CRC Failure 3"(w285) -> ()
                        n222 = local write "% Failure 3"(w285) -> ()
                      }
                      frame 3 {
                        n223 = local write "Channel 4"(w286) -> ()
                        n224 = local write "Frames Read 4"(w286) -> ()
                        n225 = local write "CRC Failure 4"(w286) -> ()
                        n226 = local write "% Failure 4"(w286) -> ()
                      }
                      frame 4 {
                        n227 = local write "Channel 5"(w287) -> ()
                        n228 = local write "Frames Read 5"(w287) -> ()
                        n229 = local write "CRC Failure 5"(w287) -> ()
                        n230 = local write "% Failure 5"(w287) -> ()
                      }
                      frame 5 {
                        n231 = local write "Channel 6"(w288) -> ()
                        n232 = local write "Frames Read 6"(w288) -> ()
                        n233 = local write "CRC Failure 5"(w288) -> ()
                        n234 = local write "% Failure 5"(w288) -> ()
                      }
                      frame 6 {
                        n235 = local write "Channel 7"(w289) -> ()
                        n236 = local write "Frames Read 7"(w289) -> ()
                        n237 = local write "CRC Failure 7"(w289) -> ()
                        n238 = local write "% Failure 7"(w289) -> ()
                      }
                      frame 7 {
                        n239 = local write "Channel 8"(w290) -> ()
                        n240 = local write "Frames Read 8"(w290) -> ()
                        n241 = local write "CRC Failure 8"(w290) -> ()
                        n242 = local write "% Failure 8"(w290) -> ()
                      }
                    }
                  }
                  n243 = local read "Configuration Folder Path"() -> (w275:path)
                  n244 = control-ref of="Port Configuration"() -> (w276:refnum<vi>)
                  n245 = control-ref of="Data Structure Folder Path"() -> (w269:refnum<vi>)
                  n246 = call "Hardware ports Config.vi"("Ring Refnum"=w276, "Configuration Folder path"=w275) -> ("data"=w271:T12)  [unwired: 9 in]
                  n247 = control-ref of="Multicolumn Listbox"() -> (w268:refnum<vi>)
                  n248 = control-ref of="FCS Configuration"() -> (w267:refnum<vi>)
                  n249 = call "Extract Frame Structure.vi"("Ring Refnum"=w267, "MCListbox Refnum"=w268, "Path in"=w269) -> ("array"=w266:string[][])  [unwired: 8 in]
                  n250 = Send Notification(notification=w271, notifier=w279) -> (notifier out=w278:refnum<notifier>, error out=w277:errorcluster)  [unwired: 1 in]
                  n251 = Bundle By Name(cluster=w272, "Port config.data"=w271, "Data Structure"=w266) -> (w270:T7)
                }
                frame "File Open" {
                  n252 = Unbundle By Name(w292) -> ("Port config.data"=w297:T12)
                  n253 = flat-sequence {
                    tunnel: w297 -> [w311]
                    tunnel: [w303] -> w294
                    tunnel: [w302] -> w293
                    tunnel: [w312] -> w299
                    tunnel: [w301] -> w298
                    tunnel: [w356] -> w295
                    tunnel: [w357] -> w296
                    tunnel: w299 -> [w357]
                    tunnel: w298 -> [w356]
                    frame #0 {
                      n254 = local read "Data Folder Path"() -> (w310:path)
                      n255 = case shown="\"bin type\", Default" "Data File Type" {
                        tunnel: [".bin" ("pattern (all files)") ".txt" ("pattern (all files)")] -> w305
                        frame "bin type", Default {
                        }
                        frame "txt type" {
                        }
                      }
                      n256 = Get Date/Time String(date format (0)=enum16{"short", "long", "abbreviated"}."abbreviated") -> (date string=w309:string)  [unwired: 2 in, 1 out]
                      n257 = Build Path(base path=w310, name or relative path=w309) -> (appended path=w308:path)
                      n258 = Create Folder(path (use dialog)=w308) -> (created path=w307:path, error out=w306:errorcluster)  [unwired: 2 in, 1 out]
                      n259 = call "File Dialog"("start path"=w307, "prompt"="Provide File Name to Save", "pattern (all files)"=w305) -> ("selected path"=w313:path)  [unwired: 9 in, 3 out]
                      n260 = call <vilib>:"Clear Errors.vi"("error in (no error)"=w306) -> ()  [unwired: 5 in, 2 out]
                      n261 = for {
                        tunnel: w311 -> [w330] mode=indexing
                        tunnel: w313 -> [w328]
                        tunnel: [w327] -> w312 mode=indexing
                        tunnel: [w325] -> w301 mode=indexing
                        tunnel: [w320] -> w303 mode=indexing
                        tunnel: [w319] -> w302 mode=indexing
                        i -> [w326]
                        n262 = case shown="2" w326 {
                          tunnel: [w331 w332 w333 w334 w335 w336 w337 w338] -> w322
                          frame 0, Default {
                            n263 = control-ref of="Channel1"() -> (w331:refnum<vi>)
                          }
                          frame 1 {
                            n264 = control-ref of="Channel2"() -> (w332:refnum<vi>)
                          }
                          frame 2 {
                            n265 = control-ref of="Channel3"() -> (w333:refnum<vi>)
                          }
                          frame 3 {
                            n266 = control-ref of="Channel4"() -> (w334:refnum<vi>)
                          }
                          frame 4 {
                            n267 = control-ref of="Channel5"() -> (w335:refnum<vi>)
                          }
                          frame 5 {
                            n268 = control-ref of="Channel6"() -> (w336:refnum<vi>)
                          }
                          frame 6 {
                            n269 = control-ref of="Channel7"() -> (w337:refnum<vi>)
                          }
                          frame 7 {
                            n270 = control-ref of="Channel8"() -> (w338:refnum<vi>)
                          }
                        }
                        n271 = control-ref of="Log CRC Failure"() -> (w318:refnum<vi>)
                        n272 = Unbundle By Name(w330) -> ("Checkbox"=w329:bool, "Port No."=w324:refnum<visa-resource-name>)
                        n273 = control-ref of="Data File Type"() -> (w323:refnum<vi>)
                        n274 = property class="Clust (strict)"(reference=w322) -> ("Label.Text"=w321:string)  [unwired: 1 in, 2 out]
                        n275 = case shown="True" w329 {
                          tunnel: [w339 w345] -> w327
                          tunnel: w321 -> [_ w347]
                          tunnel: w328 -> [w339 w346]
                          tunnel: [_ w343] -> w325
                          tunnel: w324 -> [_ _]
                          tunnel: w323 -> [_ w344]
                          tunnel: [w339 w342] -> w320
                          tunnel: [_ w341] -> w319
                          tunnel: w318 -> [_ w340]
                          frame False {
                          }
                          frame True {
                            n276 = call "File Rename.vi"("RadioBtnsControl Refnum 2"=w340, "RadioBtnsControl Refnum"=w344, "Label.Text"=w347, "selected path"=w346) -> ("CRC file refnum"=w341:refnum<file>, "CRC File Path"=w342:path, "refnum out"=w343:refnum<file>, "Path"=w345:path)  [unwired: 4 in]
                          }
                        }
                      }
                    }
                    frame #1 {
                      n277 = Get Date/Time String(want seconds? (F)=TRUE) -> (date string=w354:string, time string=w353:string)  [unwired: 2 in]
                      n278 = Concatenate Strings(w354, "   " ("string"), w353, "   " ("string"), "HOST: MSG:" ("string"), "Data Capturing Started..." ("string")) -> (w355:string)
                      n279 = local write "Status"(w355) -> ()
                    }
                  }
                  n280 = Bundle By Name(cluster=w292, "log paths"=w296, "log refnum"=w295, "CRC paths"=w294, "CRC refnum"=w293) -> (w291:T7)
                }
                frame "Process Data" {
                  n281 = Unbundle By Name(w367) -> ("Port config.data"=w369:T12, "unfiltered array"=w368:string[], "Data Structure"=w363:string[][], "CRC refnum"=w358:refnum<file>[])
                  n282 = Dequeue Element(queue=w371, timeout in ms (-1)=10) -> (element=w370:string[])  [unwired: 1 in, 3 out]
                  n283 = call <vilib>:"High Resolution Relative Seconds.vi"() -> ("relative seconds"=w362:dbl)
                  n284 = Subtract(x=w362, y=w361) -> (x-y=→"Proc loop time":dbl)
                  n285 = for {
                    tunnel: w368 -> [w382]
                    tunnel: [w383] -> w366 mode=indexing
                    tunnel: w370 -> [w380] mode=indexing
                    tunnel: w363 -> [w381]
                    tunnel: w358 -> [w377] mode=indexing
                    tunnel: [w375] -> w365 mode=indexing
                    tunnel: w369 -> [w374] mode=indexing
                    i -> [w376]
                    n286 = Unbundle By Name(w374) -> ("Checkbox"=w373:bool)
                    n287 = Index Array(array=w382, index=w376) -> (element=w378:string)
                    n288 = Concatenate Strings(w378, w380) -> (w379:string)
                    n289 = case shown="True" w373 {
                      tunnel: w381 -> [_ w394]
                      tunnel: w379 -> [w385 w395]
                      tunnel: [w385 w388] -> w383
                      tunnel: w376 -> [_ w393]
                      tunnel: w377 -> [w384 w391]
                      tunnel: [w384 w390] -> _
                      tunnel: [_ w386] -> w375
                      frame False {
                      }
                      frame True {
                        n290 = call "Process Read buffer.vi"("String Buffer"=w395, "Data Structure"=w394, "CRC file refnum"=w391) -> ("Frame Read"=w392:u32, "Filtered array"=w387:u16[], "Data Out"=w388:string, "CRC file refnum out"=w390:refnum<file>, "CRC count"=w389:u8)  [unwired: 12 in]
                        n291 = case shown="6" w393 {
                          tunnel: w392 -> [w404 w416 w428 w442 w452 w467 w479 w491]
                          tunnel: w389 -> [w396 w408 w420 w432 w444 w456 w468 w480]
                          frame 0, Default {
                            n292 = local read "CRC Failure"() -> (w399:u32)
                            n293 = To Unsigned Byte Integer(number=w404) -> (unsigned 8bit integer=w407:u8)
                            n294 = local read "Frames Read"() -> (w402:u32)
                            n295 = local read "Channel 1"() -> (w406:u8)
                            n296 = Add(x=w396, y=w399) -> (x+y=w398:u32)
                            n297 = Divide(x=w399, y=w402) -> (x/y=w401:dbl)
                            n298 = local write "CRC Failure"(w398) -> ()
                            n299 = Multiply(x=w401, y=100.0) -> (x*y=w397:dbl)
                            n300 = Add(x=w404, y=w402) -> (x+y=→"Frames Read":u32)
                            n301 = Add(x=w406, y=w407) -> (x+y=→"Channel 1":u8)
                            n302 = local write "% Failure"(w397) -> ()
                          }
                          frame 1 {
                            n303 = To Unsigned Byte Integer(number=w416) -> (unsigned 8bit integer=w419:u8)
                            n304 = local read "Frames Read 2"() -> (w414:u32)
                            n305 = local read "CRC Failure 2"() -> (w411:u32)
                            n306 = local read "Channel 2"() -> (w418:u8)
                            n307 = Add(x=w408, y=w411) -> (x+y=w410:u32)
                            n308 = Divide(x=w411, y=w414) -> (x/y=w413:dbl)
                            n309 = Add(x=w414, y=w416) -> (x+y=→"Frames Read 2":u32)
                            n310 = Add(x=w418, y=w419) -> (x+y=→"Channel 2":u8)
                            n311 = local write "CRC Failure 2"(w410) -> ()
                            n312 = Multiply(x=w413, y=100.0) -> (x*y=w409:dbl)
                            n313 = local write "% Failure 2"(w409) -> ()
                          }
                          frame 2 {
                            n314 = local read "Frames Read 3"() -> (w426:u32)
                            n315 = To Unsigned Byte Integer(number=w428) -> (unsigned 8bit integer=w431:u8)
                            n316 = local read "CRC Failure 3"() -> (w423:u32)
                            n317 = local read "Channel 3"() -> (w429:u8)
                            n318 = Add(x=w420, y=w423) -> (x+y=w422:u32)
                            n319 = Add(x=w428, y=w426) -> (x+y=→"Frames Read 3":u32)
                            n320 = Divide(x=w423, y=w426) -> (x/y=w425:dbl)
                            n321 = Add(x=w431, y=w429) -> (x+y=→"Channel 3":u8)
                            n322 = local write "CRC Failure 3"(w422) -> ()
                            n323 = Multiply(x=w425, y=100.0) -> (x*y=w421:dbl)
                            n324 = local write "% Failure 3"(w421) -> ()
                          }
                          frame 3 {
                            n325 = To Unsigned Byte Integer(number=w442) -> (unsigned 8bit integer=w443:u8)
                            n326 = local read "Frames Read 4"() -> (w438:u32)
                            n327 = local read "CRC Failure 4"() -> (w435:u32)
                            n328 = local read "Channel 4"() -> (w439:u8)
                            n329 = Add(x=w432, y=w435) -> (x+y=w434:u32)
                            n330 = Divide(x=w435, y=w438) -> (x/y=w437:dbl)
                            n331 = Add(x=w438, y=w442) -> (x+y=→"Frames Read 4":u32)
                            n332 = Add(x=w439, y=w443) -> (x+y=→"Channel 4":u8)
                            n333 = local write "CRC Failure 4"(w434) -> ()
                            n334 = Multiply(x=w437, y=100.0) -> (x*y=w433:dbl)
                            n335 = local write "% Failure 4"(w433) -> ()
                          }
                          frame 4 {
                            n336 = To Unsigned Byte Integer(number=w452) -> (unsigned 8bit integer=w455:u8)
                            n337 = local read "Frames Read 5"() -> (w450:u32)
                            n338 = local read "CRC Failure 5"() -> (w447:u32)
                            n339 = local read "Channel 5"() -> (w453:u8)
                            n340 = Add(x=w444, y=w447) -> (x+y=w446:u32)
                            n341 = Add(x=w453, y=w455) -> (x+y=→"Channel 5":u8)
                            n342 = Add(x=w450, y=w452) -> (x+y=→"Frames Read 5":u32)
                            n343 = Divide(x=w447, y=w450) -> (x/y=w449:dbl)
                            n344 = local write "CRC Failure 5"(w446) -> ()
                            n345 = Multiply(x=w449, y=100.0) -> (x*y=w445:dbl)
                            n346 = local write "% Failure 5"(w445) -> ()
                          }
                          frame 5 {
                            n347 = local read "Frames Read 6"() -> (w462:u32)
                            n348 = local read "CRC Failure 6"() -> (w459:u32)
                            n349 = To Unsigned Byte Integer(number=w467) -> (unsigned 8bit integer=w466:u8)
                            n350 = local read "Channel 6"() -> (w464:u8)
                            n351 = Add(x=w456, y=w459) -> (x+y=w458:u32)
                            n352 = Add(x=w462, y=w467) -> (x+y=→"Frames Read 6":u32)
                            n353 = Divide(x=w459, y=w462) -> (x/y=w461:dbl)
                            n354 = Add(x=w466, y=w464) -> (x+y=→"Channel 6":u8)
                            n355 = local write "CRC Failure 6"(w458) -> ()
                            n356 = Multiply(x=w461, y=100.0) -> (x*y=w457:dbl)
                            n357 = local write "% Failure 6"(w457) -> ()
                          }
                          frame 6 {
                            n358 = local read "Frames Read 7"() -> (w474:u32)
                            n359 = To Unsigned Byte Integer(number=w479) -> (unsigned 8bit integer=w478:u8)
                            n360 = local read "CRC Failure 7"() -> (w471:u32)
                            n361 = local read "Channel 7"() -> (w475:u8)
                            n362 = Add(x=w474, y=w479) -> (x+y=→"Frames Read 7":u32)
                            n363 = Add(x=w468, y=w471) -> (x+y=w470:u32)
                            n364 = Add(x=w475, y=w478) -> (x+y=→"Channel 7":u8)
                            n365 = Divide(x=w471, y=w474) -> (x/y=w473:dbl)
                            n366 = local write "CRC Failure 7"(w470) -> ()
                            n367 = Multiply(x=w473, y=100.0) -> (x*y=w469:dbl)
                            n368 = local write "% Failure 7"(w469) -> ()
                          }
                          frame 7 {
                            n369 = local read "Frames Read 8"() -> (w486:u32)
                            n370 = local read "Channel 8"() -> (w487:u8)
                            n371 = To Unsigned Byte Integer(number=w491) -> (unsigned 8bit integer=w490:u8)
                            n372 = local read "CRC Failure 8"() -> (w483:u32)
                            n373 = Add(x=w487, y=w490) -> (x+y=→"Channel 8":u8)
                            n374 = Add(x=w480, y=w483) -> (x+y=w482:u32)
                            n375 = Divide(x=w483, y=w486) -> (x/y=w485:dbl)
                            n376 = Add(x=w491, y=w486) -> (x+y=→"Frames Read 8":u32)
                            n377 = local write "CRC Failure 8"(w482) -> ()
                            n378 = Multiply(x=w485, y=100.0) -> (x*y=w481:dbl)
                            n379 = local write "% Failure 8"(w481) -> ()
                          }
                        }
                        n380 = Byte Array To String(unsigned byte array=w387) -> (string=w386:string)
                      }
                    }
                  }
                  n381 = Bundle By Name(cluster=w367, "unfiltered array"=w366, "Filtered array"=w365) -> (w364:T7)
                }
                frame "Data Logging" {
                  n382 = Unbundle By Name(w493) -> ("Filtered array"=w494:string[], "log refnum"=w495:refnum<file>[])
                  n383 = local read "Data File Type"() -> (w496:enum32{"bin type", "txt type"})
                  n384 = for {
                    tunnel: w495 -> [w502] mode=indexing
                    tunnel: w494 -> [w498] mode=indexing
                    tunnel: w496 -> [w499]
                    n385 = String To Byte Array(string=w498) -> (unsigned byte array=w501:u8[])
                    n386 = Empty Array?(array=w501) -> (empty?=w500:bool)
                    n387 = case shown="False" w500 {
                      tunnel: w502 -> [w507 w522]
                      tunnel: [w506 w522] -> _
                      tunnel: w501 -> [w505 _]
                      tunnel: w499 -> [w504 _]
                      tunnel: w498 -> [w503 _]
                      frame False {
                        n388 = case shown="\"txt type\"" w504 {
                          tunnel: w507 -> [w510 w513]
                          tunnel: [w509 w512] -> w506
                          tunnel: w505 -> [_ w514]
                          tunnel: w503 -> [w511 _]
                          frame "bin type", Default {
                            n389 = Write to Binary File(file (use dialog)=w510, data=w511, 9:T10."little-endian" ("byte order (0:big-endian, network order)")) -> (refnum out=w509:refnum<file>)  [unwired: 3 in, 2 out]
                          }
                          frame "txt type" {
                            n390 = for {
                              tunnel: w514 -> [w521] mode=indexing
                              shift-right: [w515] -> w512
                              shift-left: w513 -> [w516]
                              n391 = Format Into String(format string="%x", w521) -> (resulting string=w519:string)  [unwired: 2 in, 1 out]
                              n392 = call <vilib>:"Space Constant.vi"() -> ("String"=w518:string)
                              n393 = Concatenate Strings(w519, w518) -> (w517:string)
                              n394 = Write to Text File(file (use dialog)=w516, text=w517) -> (refnum out=w515:refnum<file>)  [unwired: 2 in, 2 out]
                            }
                          }
                        }
                      }
                      frame True {
                      }
                    }
                  }
                }
                frame "File Close" {
                  n395 = Unbundle By Name(w525) -> ("Port config.data"=w524:T12, "log paths"=w529:path[], "log refnum"=w528:refnum<file>[], "CRC refnum"=w527:refnum<file>[], "CRC paths"=w526:path[])
                  n396 = Send Notification(notification="Stop Acquisition", notifier=w533) -> (notifier out=w531:refnum<notifier>, error out=w530:errorcluster)  [unwired: 1 in]
                  n397 = case shown="True" "Stop Acquisition" {
                    tunnel: w528 -> [_ w543]
                    tunnel: [w538 w542] -> _
                    tunnel: w529 -> [w538 _]
                    tunnel: w527 -> [_ w540]
                    tunnel: w526 -> [w537 _]
                    tunnel: [w537 w541] -> _
                    tunnel: w524 -> [_ w539]
                    frame False {
                    }
                    frame True {
                      n398 = for {
                        tunnel: [w552] -> _ mode=indexing
                        tunnel: w543 -> [w551] mode=indexing
                        tunnel: [w550] -> w542 mode=indexing
                        tunnel: [w549] -> _ mode=indexing
                        tunnel: [w547] -> w541 mode=indexing
                        tunnel: w540 -> [w548] mode=indexing
                        tunnel: [w546] -> _ mode=indexing
                        tunnel: w539 -> [w545] mode=indexing
                        n399 = Unbundle By Name(w545) -> ("Port No."=w544:refnum<visa-resource-name>)
                        n400 = Close File(refnum=w551) -> (path=w550:path, error out=w549:errorcluster)  [unwired: 1 in]
                        n401 = Close File(refnum=w548) -> (path=w547:path, error out=w546:errorcluster)  [unwired: 1 in]
                        n402 = VISA Close(VISA resource name=w544) -> (error out=w552:errorcluster)  [unwired: 1 in]
                      }
                    }
                  }
                  n403 = Select(t=Data_Acquisition."Exit", s="Stop Acquisition", f=Data_Acquisition."Process Data") -> (s? t:f=w535:T9)
                }
                frame "Exit" {
                  n404 = Get Date/Time String(want seconds? (F)=TRUE) -> (date string=w563:string, time string=w564:string)  [unwired: 2 in]
                  n405 = Concatenate Strings(w563, "   " ("string"), w564, "   " ("string"), "HOST: MSG:" ("string"), "Stopped!!!" ("string")) -> (w562:string)
                  n406 = local write "Status"(w562) -> ()
                }
              }
              n407 = control-ref of="Stop Acquisition"() -> (w264:refnum<vi>)
              n408 = property class="Bool"(reference=w264, "DisabledEnum"=T6."Enabled" ("Disabled")) -> ()  [unwired: 1 in, 2 out]
              n409 = control-ref of="Start Acquisition"() -> (w263:refnum<vi>)
              n410 = property class="Bool"(reference=w263, "DisabledEnum"=T6."Disabled and Grayed Out" ("Disabled")) -> ()  [unwired: 1 in, 2 out]
            }
            n411 = Wait on Notification(notifier=w244, ignore previous (F)=TRUE) -> (notification=w230:T8)  [unwired: 2 in, 3 out]
            n412 = call "Raw data read Parallel.vi"("error in (no error)"=w229, "Data Queue in"=w232, "notifier in"=w231, "Array"=w230) -> ("error out"=w228:errorcluster, "Data queue out"=w227:refnum<queue>)  [unwired: 6 in]
            n413 = Release Queue(queue=w227, error in (no error)=w228) -> ()  [unwired: 1 in, 3 out]
            n414 = Release Notifier(notifier=w243, error in (no error)=w241) -> ()  [unwired: 1 in, 3 out]
            n415 = Release Notifier(notifier=w237, error in (no error)=w236) -> ()  [unwired: 1 in, 3 out]
          }
        }
        n416 = control-ref of="Stop Acquisition"() -> (w219:refnum<vi>)
        n417 = property class="Bool"(reference=w219, "DisabledEnum"=T6."Disabled and Grayed Out" ("Disabled")) -> ()  [unwired: 1 in, 2 out]
        n418 = control-ref of="Start Acquisition"() -> (w217:refnum<vi>)
        n419 = property class="Bool"(reference=w217, "DisabledEnum"=T6."Enabled" ("Disabled")) -> ()  [unwired: 1 in, 2 out]
        n420 = control-ref of="FCS Configuration"() -> (w221:refnum<vi>)
        n421 = control-ref of="Configuration Folder Path"() -> (w223:refnum<vi>)
        n422 = control-ref of="Data Structure Folder Path"() -> (w224:refnum<vi>)
        n423 = control-ref of="Port Configuration"() -> (w222:refnum<vi>)
        n424 = call "Config select.vi"("Ring Refnum 2"=w221, "Ring Refnum"=w222, "reference in"=w223, "Path in"=w224) -> ()  [unwired: 8 in]
        n425 = property class="VI"("Front Panel.Title"="FCS Test Jig - Acquisition Panel" ("VI Name")) -> ()  [unwired: 2 in, 2 out]
      }
      frame "Configuration" {
        n426 = case shown="True" "Update" {
          tunnel: w567 -> [w572 w590]
          tunnel: [w572 w584] -> _
          frame False {
          }
          frame True {
            w580 = "\t"
            n427 = call <vilib>:"Application Directory.vi"() -> ("Application Directory"=w582:path)
            n428 = local read "Data File Type"() -> (w579:enum32{"bin type", "txt type"})
            n429 = Build Path(base path=w582, name or relative path="File Paths.txt") -> (appended path=w581:path)
            n430 = Format Into String(w579) -> (resulting string=w578:string)  [unwired: 3 in, 1 out]
            n431 = Format Into String("Log CRC Failure") -> (resulting string=w577:string)  [unwired: 3 in, 1 out]
            n432 = Format Into String("Configuration Folder Path", "\t", "Data Structure Folder Path", w580, "Data Folder Path", w580, w578, w580, w577) -> (resulting string=w587:string)  [unwired: 3 in, 1 out]
            n433 = Open/Create/Replace File(file path (use dialog)=w581, error in=w590, operation (0:open)=T11."replace or create") -> (refnum out=w588:refnum<file>, error out=w589:errorcluster)  [unwired: 3 in, 1 out]
            n434 = Write to Text File(file (use dialog)=w588, text=w587, error in=w589) -> (refnum out=w585:refnum<file>, error out=w586:errorcluster)  [unwired: 1 in, 1 out]
            n435 = Close File(refnum=w585, error in=w586) -> (error out=w584:errorcluster)  [unwired: 1 out]
          }
        }
        n436 = case shown="True" "Done" {
          frame False {
          }
          frame True {
            n437 = local write "Tab Control"(T1."Home" ("Tab Control")) -> ()
            n438 = property class="VI"("Front Panel.Title"="FCS Test Jig - Home Page" ("VI Name")) -> ()  [unwired: 2 in, 2 out]
          }
        }
        n439 = property class="VI"("Front Panel.Title"="FCS Test Jig - Settings Panel" ("VI Name")) -> ()  [unwired: 2 in, 2 out]
      }
      frame "User Info" {
        n440 = control-ref of="Add user"() -> (w599:refnum<vi>)
        n441 = control-ref of="Delete User"() -> (w598:refnum<vi>)
        n442 = control-ref of="View users"() -> (w597:refnum<vi>)
        n443 = control-ref of="User Name"() -> (w594:refnum<vi>)
        n444 = control-ref of="Password"() -> (w603:refnum<vi>)
        n445 = control-ref of="User Name"() -> (w593:refnum<vi>)
        n446 = call "Admin Options.vi"("reference"=w593, "View users"=w597, "Delete User"=w598, "Boolean in"=w599) -> ()  [unwired: 8 in]
        n447 = control-ref of="Signin"() -> (w606:refnum<vi>)
        n448 = control-ref of="User Name"() -> (w595:refnum<vi>)
        n449 = control-ref of="Password"() -> (w609:refnum<vi>)
        n450 = control-ref of="login text"() -> (w608:refnum<vi>)
        n451 = call "Password Change.vi"("Confirm"="Confirm", "New Password"="New Password", "Current Password"="Current Password", "reference in"=w594, "String in"=w603) -> ("Success"=→"Success":string)  [unwired: 6 in]
        n452 = Build Array(w595, w609, w608, w606) -> (w607:refnum<vi>[])
        n453 = for {
          tunnel: w607 -> [w623] mode=indexing
          tunnel: [w622] -> _ mode=indexing
          w628 = refnum<vi> refnum  # Control
          n454 = To More Generic Class(target class=w628, reference=w623) -> (generic class reference=w627:refnum<vi>)
          n455 = property class="Ctl"(reference=w627, "Visible"=FALSE) -> (reference out=w625:refnum<vi>, error out=w626:errorcluster)  [unwired: 1 in]
          n456 = Close Reference(reference=w625, error in (no error)=w626) -> (error out=w622:errorcluster)
        }
        n457 = case shown="True" "Change password" {
          frame False {
          }
          frame True {
            n458 = control-ref of="Confirm"() -> (w611:refnum<vi>)
            n459 = control-ref of="New Password"() -> (w613:refnum<vi>)
            n460 = control-ref of="Current Password"() -> (w612:refnum<vi>)
            n461 = control-ref of="Success"() -> (w610:refnum<vi>)
            n462 = Build Array(w613, w612, w611, w610) -> (w614:refnum<vi>[])
            n463 = for {
              tunnel: w614 -> [w616] mode=indexing
              tunnel: [w615] -> _ mode=indexing
              w621 = refnum<vi> refnum  # Control
              n464 = To More Generic Class(target class=w621, reference=w616) -> (generic class reference=w620:refnum<vi>)
              n465 = property class="Ctl"(reference=w620, "Visible"=TRUE) -> (reference out=w618:refnum<vi>, error out=w619:errorcluster)  [unwired: 1 in]
              n466 = Close Reference(reference=w618, error in (no error)=w619) -> (error out=w615:errorcluster)
            }
          }
        }
      }
      frame "Logout" {
        n467 = Format Into String(w629, " has logged out successfully!" ("String")) -> (resulting string=w630:string)  [unwired: 3 in, 1 out]
        n468 = Get Date/Time String(want seconds? (F)=TRUE) -> (date string=w637:string, time string=w638:string)  [unwired: 2 in]
        n469 = Concatenate Strings(w637, "          ", w638, "          ", "HOST: MSG: " ("string"), w630) -> (w632:string)
        n470 = local write "Status"(w632) -> ()
      }
      frame "Exit" {
      }
    }
  }
  "error out" <- w2
  n471 = disable-structure shown="Disabled" {
    frame Disabled {
      n472 = while {
        tunnel: _ -> [w653]
        tunnel: [w652] -> _
        tunnel: [w651] -> _
        tunnel: _ -> [w650]
        tunnel: _ -> [w649]
        tunnel: _ -> [w647]
        tunnel: _ -> [w646]
        stop <- w648 stop-if-true
        n473 = Wait on Notification(notifier=w647, ignore previous (F)=TRUE, timeout in ms (-1)=10, error in (no error)=w646) -> (notification=w648:bool)  [unwired: 3 out]
        n474 = for {
          tunnel: w649 -> [w657] mode=indexing
          tunnel: [w656] -> w654 mode=indexing
          workers-P: 8 -> [_]
          n475 = Unbundle By Name(w657) -> ("Port No."=w658, "Checkbox"=w655)
          n476 = case shown="True" w655 {
            tunnel: w658 -> [_ w662]
            tunnel: [_ w664] -> w656
            tunnel: [_ w663] -> _
            frame False {
            }
            frame True {
              n477 = property class="Instr"(reference=w662) -> (reference out=w661:refnum<visa-resource-name>, "Bytes at Port"=w660:u32)  [unwired: 1 in, 1 out]
              n478 = Greater Than 0?(x=w660) -> (x > 0?=w659:bool)
              n479 = case shown="True" w659 {
                tunnel: w661 -> [w665 w670]
                tunnel: [_ w668] -> w664
                tunnel: [_ w669] -> w663
                tunnel: w660 -> [_ w666]
                tunnel: [w665 w667] -> _
                frame False {
                }
                frame True {
                  n480 = VISA Read(VISA resource name=w670, byte count=w666) -> (VISA resource name out=w667:refnum<visa-resource-name>, read buffer=w668:string, error out=w669:errorcluster)  [unwired: 1 in, 1 out]
                }
              }
            }
          }
        }
        n481 = Enqueue Element(queue=w653, element=w654, timeout in ms (-1)=10, error in (no error)=w650) -> (queue out=w652:refnum<queue>, error out=w651:errorcluster)  [unwired: 1 out]
      }
    }
    frame Enabled {
    }
  }
